vi "_Veritech_LVCM_Global_OnCommand.vi"(10 "Command ID":string, 11 "Object":T1) -> ()   [LabVIEW 2014]
uses:
  <resource>/Framework/Providers/API/ItemRef.ctl
  <vilib>/dlg_ctls.llb/Space Constant.vi
  Support/Utilites/GCMLog/LogInfo.vi
  Support/Framework/ItemSelection/ItemSelection.lvlib
  Support/Utilites/GCMLog/GCMLog.lvclass
panel:
  out "error out":errorcluster
  in  "error in":errorcluster
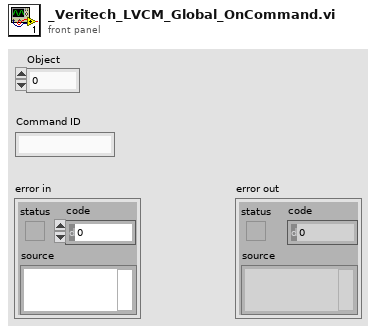
[diagram p1: front panel]
types:
  T1 = typedef "ItemRef.ctl" = u64
  T2 = cluster{"Item URL":string, "Item ID":string, "Item Index":i32, "Specific Type":string}
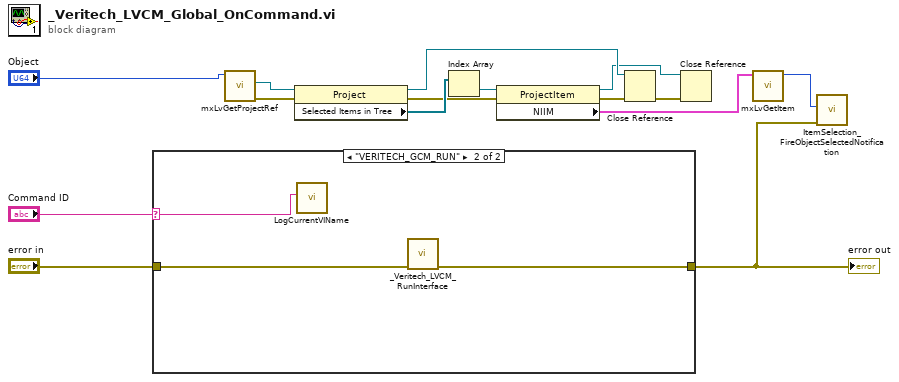
[diagram p0: block diagram]
diagram:
  n1 = case shown="\"VERITECH_GCM_RUN\"" "Command ID" {
    selector: "Command ID" -> [_ w19]
    tunnel: "error in" -> [w16 w18]
    tunnel: [w16 w17] -> w9
    frame Default {
    }
    frame "VERITECH_GCM_RUN" {
      n2 = call "LogCurrentVIName.vi"("AdditionalInfo"=w19) -> ()  [unwired: 10 in, 1 out]
      n3 = call "_Veritech_LVCM_RunInterface.vi"("error in (no error)"=w18) -> ("error out"=w17:errorcluster)  [unwired: 10 in]
    }
  }
  "error out" <- w9
  n4 = call <resource>:"mxLvGetProjectRef.vi"("Item"="Object") -> ("error out"=w11:errorcluster, "Project Refnum"=w12:refnum<vi>)  [unwired: 8 in, 1 out]
  n5 = property class="Project"(reference=w12, error in=w11) -> (reference out=w3:refnum<vi>, error out=w5:errorcluster, "Selected Items in Tree"=w10:refnum<vi>[])
  n6 = Index Array(array=w10) -> (element=w7:refnum<vi>)  [unwired: 1 in]
  n7 = property class="ProjectItem"(reference=w7, error in=w5) -> (reference out=w1:refnum<vi>, error out=w4:errorcluster, "NIIM"=w6:T2)
  n8 = Close Reference(reference=w3, error in (no error)=w4) -> (error out=w2:errorcluster)
  n9 = Close Reference(reference=w1, error in (no error)=w2) -> ()  [unwired: 1 out]
  n10 = call <resource>:"mxLvGetItem.vi"("NIIM"=w6) -> ("Item"=w8:T1)  [unwired: 9 in, 1 out]
  n11 = call "ItemSelection_FireObjectSelectedNotification.vi"("error in (no error)"=w9, "Item Ref"=w8) -> ()  [unwired: 9 in, 1 out]
